vi "GearAiming.vi"() -> (2 "Drive Rotate":dbl, 3 "Drive Y":dbl)   [LabVIEW 2016]
uses:
  <vilib>/Rock Robotics/Network Tables/NT Read Number.vi
  <vilib>/Rock Robotics/Network Tables/NT Read Numeric Array.vi
  Robot Global Data.vi
  <vilib>/addons/control/pid/pid.llb/PID (DBL).vi
  <vilib>/addons/control/pid/NI_PID_pid.lvlib
panel:
  in  "TurnOff":dbl=29.0
  in  "Fast speed":dbl=-0.3 format="%#_13g"
  in  "Approach Speed":dbl=-0.12 format="%#_13g"
  in  "PID gains":T1={"proportional gain (Kc)"=0.019, "integral time (Ti, min)"=0.0, "derivative time (Td, min)"=0.0} {"derivative time (Td, min)" format="%.3f"; "integral time (Ti, min)" format="%.3f"; "proportional gain (Kc)" format="%.3f"}
  in  "setpoint":dbl=1400.0 format="%#_13g"
  # "Practice Bot\nP: 0.017\nI: 0\nD: 0"
  # "First District 11-2:00\nP: 0.019\nI: 0\nD: 0"
  # "\"setpoint\" Previous value: 305\nJohn changed to 1300 on 3/2"
  # "Deprecated\nMoved to Dashboard"
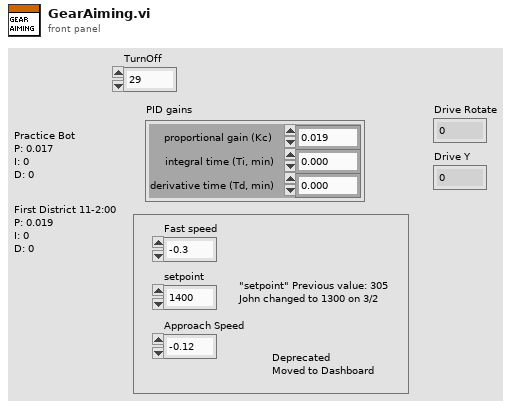
[diagram p1: front panel]
types:
  T1 = cluster{"proportional gain (Kc)":dbl, "integral time (Ti, min)":dbl, "derivative time (Td, min)":dbl}
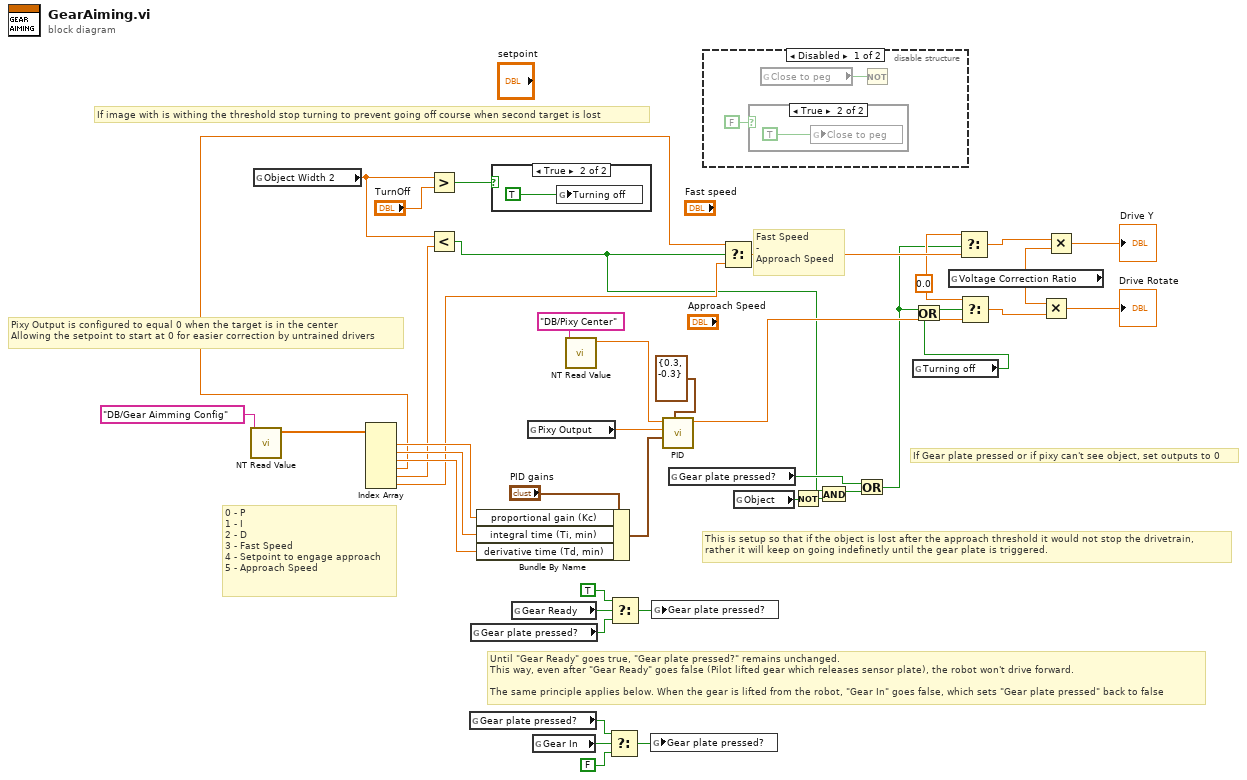
[diagram p0: block diagram]
diagram:
  w34 = 0.0 ("t")
  # "This is setup so that if the object is lost after the approach threshold it would not stop the drivetrain,\nrather it will keep on going indefinetly until the gear plate is triggered."
  # "If image with is withing the threshold stop turning to prevent going off course when second target is lost"
  # "Pixy Output is configured to equal 0 when the target is in the center\nAllowing the setpoint to start at 0 for easier correction by untrained drivers"
  # "0 - P\n1 - I\n2 - D\n3 - Fast Speed\n4 - Setpoint to engage approach\n5 - Approach Speed"
  # "Fast Speed\n-\nApproach Speed"
  # "Until \"Gear Ready\" goes true, \"Gear plate pressed?\" remains unchanged.\nThis way, even after \"Gear Ready\" goes false (Pilot lifted gear which releases sensor plate), the robot won't drive forward.\n\nThe same principle applies below. When the gear is lifted from the robot, \"Gear In\" goes false, which sets \"Gear plate pressed\" back to false"
  # "If Gear plate pressed or if pixy can't see object, set outputs to 0"
  n1 = call-poly <vilib>:"NT Read Value.vi"("Name"="DB/Gear Aimming Config") -> ("Numeric Array"=w21:dbl[])  [unwired: 9 in, 1 out]
  n2 = global read "Robot Global Data.vi" "Object Width 2"() -> (w10:dbl)
  n3 = Index Array(array=w21) -> (element #1=w18:dbl, element #2=w17:dbl, element #3=w16:dbl, element #4=w14:dbl, element #5=w13:dbl, element #6=w15:dbl)  [unwired: 6 in]
  n4 = Greater?(x=w10, y="TurnOff") -> (0:w11:bool)
  n5 = Less?(x=w10, y=w13) -> (x < y?=w5:bool)
  n6 = global read "Robot Global Data.vi" "Gear plate pressed?"() -> (w23:bool)
  n7 = global read "Robot Global Data.vi" "Gear plate pressed?"() -> (w27:bool)
  n8 = Bundle By Name(cluster="PID gains", "proportional gain (Kc)"=w18, "integral time (Ti, min)"=w17, "derivative time (Td, min)"=w16) -> (w20:T1)
  n9 = case shown="True" w11 {
    frame False {
    }
    frame True {
      n10 = global write "Robot Global Data.vi" "Turning off"(TRUE ("Close")) -> ()
    }
  }
  n11 = global read "Robot Global Data.vi" "Gear Ready"() -> (w30:bool)
  n12 = global read "Robot Global Data.vi" "Pixy Output"() -> (w35:dbl)
  n13 = global read "Robot Global Data.vi" "Gear In"() -> (w26:bool)
  n14 = call-poly <vilib>:"NT Read Value.vi"("Name"="DB/Pixy Center") -> ("Numeric"=w39:dbl)  [unwired: 9 in, 1 out]
  n15 = Select(t=w23, s=w26, f=FALSE) -> (s? t:f=w25:bool)
  n16 = Select(t=TRUE, s=w30, f=w27) -> (s? t:f=w28:bool)
  n17 = global write "Robot Global Data.vi" "Gear plate pressed?"(w25) -> ()
  n18 = global write "Robot Global Data.vi" "Gear plate pressed?"(w28) -> ()
  n19 = call-poly <vilib>:"PID.vi"("output range"=cluster{"output high":dbl, "output low":dbl} {"output high"=0.3, "output low"=-0.3}, "PID gains"=w20, "process variable"=w35, "setpoint"=w39) -> ("output"=w36:dbl)  [unwired: 6 in, 1 out]
  n20 = global read "Robot Global Data.vi" "Gear plate pressed?"() -> (w31:bool)
  n21 = disable-structure shown="Disabled" {
    frame Disabled {
      n22 = case shown="True" FALSE {
        frame False {
        }
        frame True {
          n23 = global write "Robot Global Data.vi" "Close to peg"(TRUE ("Close")) -> ()
        }
      }
      n24 = global read "Robot Global Data.vi" "Close to peg"() -> (w44:bool)
      n25 = Not(x=w44) -> ()  [unwired: 1 out]
    }
    frame Enabled {
    }
  }
  n26 = Select(t=w14, s=w5, f=w15) -> (s? t:f=w41:dbl)
  n27 = global read "Robot Global Data.vi" "Object"() -> (w33:bool)
  n28 = Not(x=w33) -> (.not. x?=w32:bool)
  n29 = And(x=w5, y=w32) -> (x .and. y?=w6:bool)
  n30 = Or(x=w31, y=w6) -> (x .or. y?=w12:bool)
  n31 = global read "Robot Global Data.vi" "Turning off"() -> (w7:bool)
  n32 = Or(x=w12, y=w7) -> (x .or. y?=w8:bool)
  n33 = global read "Robot Global Data.vi" "Voltage Correction Ratio"() -> (w1:dbl)
  n34 = Select(t=w34, s=w12, f=w41) -> (s? t:f=w2:dbl)
  n35 = Select(t=w34, s=w8, f=w36) -> (s? t:f=w40:dbl)
  n36 = Multiply(x=w1, y=w40) -> (x*y=→"Drive Rotate":dbl)
  n37 = Multiply(x=w2, y=w1) -> (x*y=→"Drive Y":dbl)
